vi "结构.vi"() -> ()   [LabVIEW 2014]
panel:
  in  "清空":bool
  out "数值 2":dbl
  in  "事件结构测试按钮":bool
  out "while":i32
  out "指示灯":bool
  out "数值":i32
  out "波形图表 2":dbl(graph)
  out "波形图表":dbl(graph)
  out "次数":i32
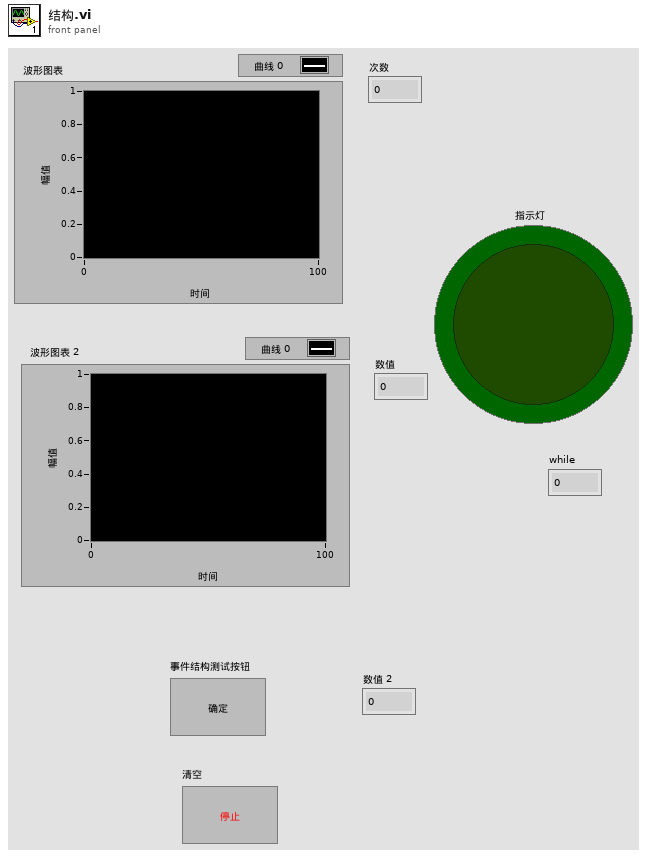
[diagram p1: front panel]
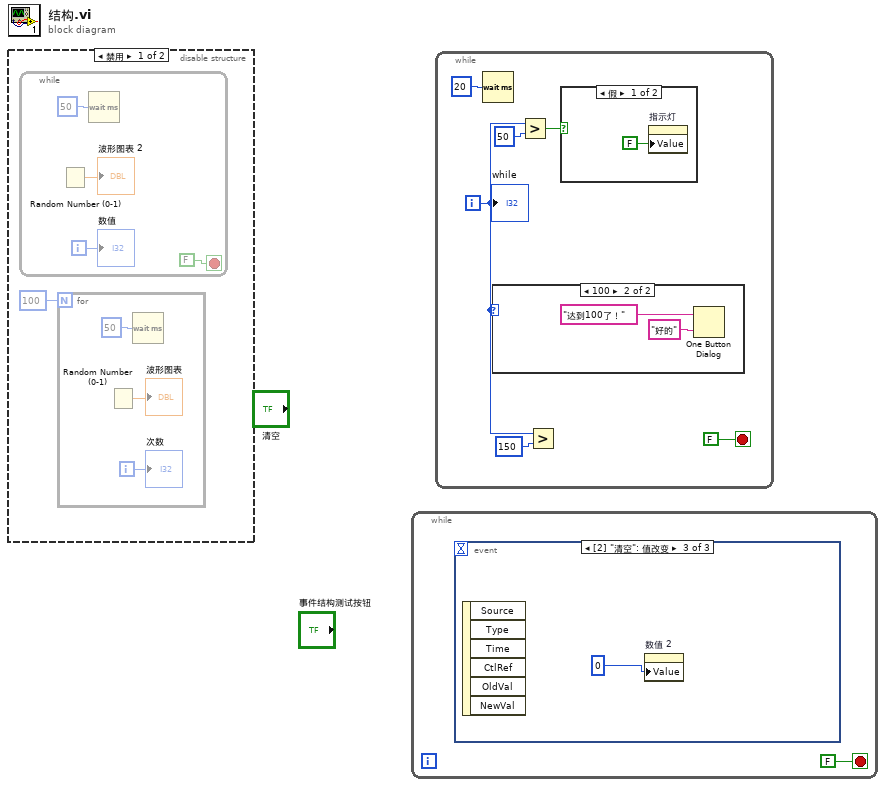
[diagram p0: block diagram]
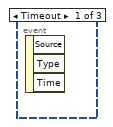
[diagram p2: hidden frame]
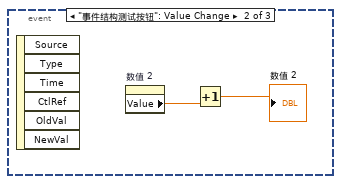
[diagram p3: hidden frame]
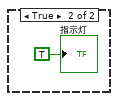
[diagram p6: hidden frame]
diagram:
  n1 = disable-structure shown="禁用" {
    frame Disabled {
      n2 = while {
        i -> [w2]
        stop <- FALSE stop-if-true
        n3 = Random Number (0-1)() -> (number: 0 to 1=→"波形图表 2":dbl)
        n4 = Wait (ms)(milliseconds to wait=u32 50 ("毫秒计时值")) -> ()  [unwired: 1 out]
        "数值" <- w2
      }
      n5 = for {
        N: 100 -> [_]
        i -> [w8]
        n6 = Random Number (0-1)() -> (number: 0 to 1=→"波形图表":dbl)
        n7 = Wait (ms)(milliseconds to wait=u32 50 ("毫秒计时值")) -> ()  [unwired: 1 out]
        "次数" <- w8
      }
    }
    frame Enabled {
    }
  }
  n8 = while {
    stop <- FALSE stop-if-true
    n9 = event shown="[2] \"清空\": 值改变" {
      selector: _ -> [_ _ _]
      dyn-events: _ -> [_ _ _]
      timeout: _ -> [_ _ _]
      event Timeout {
        n10 = event-data() -> ()  [unwired: 1 in, 3 out]
      }
      event "事件结构测试按钮": Value Change {
        n11 = event-data() -> ()  [unwired: 1 in, 6 out]
        n12 = property on="数值 2" class="DigNum (严格)"() -> ("Value"=w11:dbl)  [unwired: 2 in, 2 out]
        n13 = Increment(x=w11) -> (x+1=→"数值 2":dbl)
      }
      event "清空": Value Change {
        n14 = event-data() -> ()  [unwired: 1 in, 6 out]
        n15 = property on="数值 2" class="DigNum (严格)"("Value"=0) -> ()  [unwired: 2 in, 2 out]
      }
    }
  }
  n16 = while {
    i -> [w14]
    stop <- FALSE stop-if-true
    n17 = Wait (ms)(milliseconds to wait=u32 20 ("毫秒计时值")) -> ()  [unwired: 1 out]
    n18 = case shown="100" w14 {
      frame 0, Default {
      }
      frame 100 {
        n19 = One Button Dialog(message="达到100了！" ("消息"), button name ("OK")="好的" ("按钮名称（“确定”）")) -> ()  [unwired: 1 out]
      }
    }
    n20 = Greater?(x=w14, y=50) -> (0:w17:bool)
    n21 = Greater?(x=w14, y=150) -> ()  [unwired: 1 out]
    n22 = case shown="假" w17 {
      frame False {
        n23 = property on="指示灯" class="Bool (严格)"("Value"=FALSE ("指示灯")) -> ()  [unwired: 2 in, 2 out]
      }
      frame True {
        "指示灯" <- TRUE ("指示灯")
      }
    }
    "while" <- w14
  }
